vi "JoystickToPoint.vi"(8 "Yw":dbl, 9 "Xw":dbl, 11 "JoystickIn":i32[](array[numeric])) -> (2 "y":dbl, 3 "x":dbl)   [LabVIEW 2013, in "ProcessorHelperFunctions.lvlib"]
uses:
  ProcessorHelperFunctions.lvlib
  <vilib>/Analysis/coordinate.llb/Angle Range (Degree).ctl
  <vilib>/Analysis/coordinate.llb/Angle Rotation (scalar).vi
  <vilib>/Analysis/coordinate.llb/Wrap Angle (scalar).vi
  <vilib>/Analysis/NI_AAL_Angle.lvlib
panel:
  in  "Mag Scaler":dbl=1.5
  # "Xw is x distance between the\nwheels on the robot"
  # "Yw is y distance between the\nwheels on the robot"
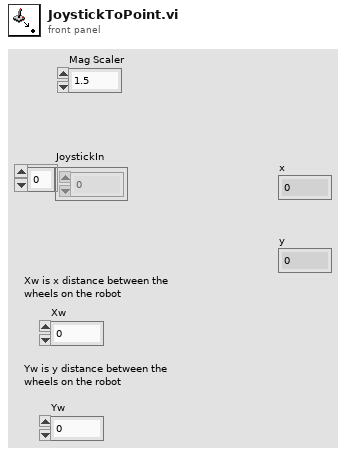
[diagram p1: front panel]
types:
  T1 = typedef "NI_AAL_Angle.lvlib/Angle Range (Degree).ctl" = u16
  T2 = cluster{"JoystickIn[0]":i32, "JoystickIn[1]":i32, "JoystickIn[2]":i32, "JoystickIn[3]":i32, "JoystickIn[4]":i32, "JoystickIn[5]":i32, "JoystickIn[6]":i32, "JoystickIn[7]":i32, "JoystickIn[8]":i32, "JoystickIn[9]":i32}
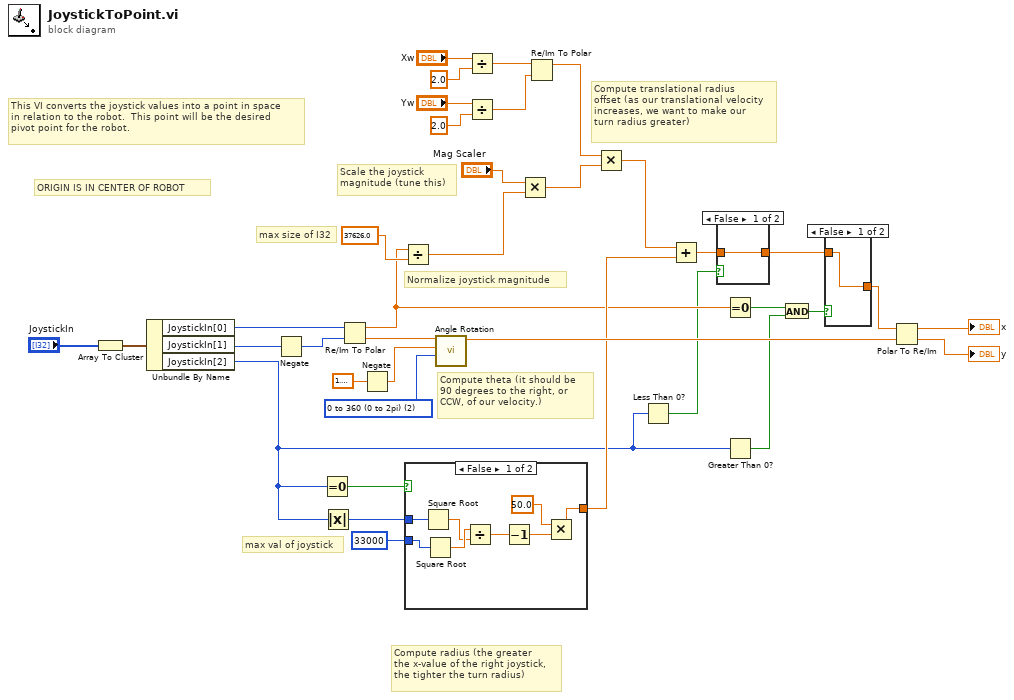
[diagram p0: block diagram]
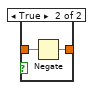
[diagram p2: hidden frame]
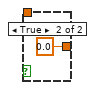
[diagram p3: hidden frame]
diagram:
  w32 = T1 2 items=["none", "-180 to 180 (-pi to pi)", "0 to 360 (0 to 2pi)"] ("rotated angle range")
  # "ORIGIN IS IN CENTER OF ROBOT"
  # "Scale the joystick\nmagnitude (tune this)"
  # "Compute theta (it should be \n90 degrees to the right, or \nCCW, of our velocity.)"
  # "Compute radius (the greater\nthe x-value of the right joystick,\nthe tighter the turn radius)"
  # "Compute translational radius \noffset (as our translational velocity\nincreases, we want to make our\nturn radius greater)"
  # "Normalize joystick magnitude"
  # "max size of I32"
  # "max val of joystick"
  # "This VI converts the joystick values into a point in space\nin relation to the robot.  This point will be the desired\npivot point for the robot."
  n1 = Array To Cluster(array="JoystickIn") -> (cluster=w37:T2)
  n2 = Unbundle By Name(w37) -> ("JoystickIn[0]"=w35:i32, "JoystickIn[1]"=w34:i32, "JoystickIn[2]"=w3:i32)
  n3 = Negate(x=w34) -> (-x=w1:i32)
  n4 = Equal To 0?(x=w3) -> (x = 0?=w30:bool)
  n5 = Absolute Value(x=w3) -> (abs(x)=w6:i32)
  n6 = Re/Im To Polar(2:w1, 3:w35) -> (0:w33:dbl, 1:w9:dbl)
  n7 = Negate(x=1.5707963267948966) -> (-x=w7:dbl)
  n8 = Divide(x=w9, y=37626.0) -> (x/y=w25:dbl)
  n9 = case shown="False" w30 {
    tunnel: 33000 -> [w44 w46]
    tunnel: w6 -> [w45 _]
    tunnel: [w40 w46] -> w21
    frame False {
      n10 = Square Root(x=w45) -> (sqrt(x)=w42:dbl)
      n11 = Square Root(x=w44) -> (sqrt(x)=w43:dbl)
      n12 = Divide(x=w43, y=w42) -> (x/y=w39:dbl)
      n13 = Decrement(x=w39) -> (x-1=w38:dbl)
      n14 = Multiply(x=50.0, y=w38) -> (x*y=w40:dbl)
    }
    frame True {
    }
  }
  n15 = call-poly <vilib>:"Angle Rotation.vi"("rotated angle range"=w32, "counterclockwise rotation"=w7, "angle"=w33) -> ("rotated angle"=w28:dbl)  [unwired: 7 in, 1 out]
  n16 = Divide(x="Xw", y=2.0) -> (x/y=w16:dbl)
  n17 = Divide(x="Yw", y=2.0) -> (x/y=w15:dbl)
  n18 = Multiply(x="Mag Scaler", y=w25) -> (x*y=w24:dbl)
  n19 = Re/Im To Polar(2:w15, 3:w16) -> (1:w23:dbl)  [unwired: 1 out]
  n20 = Multiply(x=w23, y=w24) -> (x*y=w22:dbl)
  n21 = Less Than 0?(x=w3) -> (x < 0?=w2:bool)
  n22 = Add(x=w22, y=w21) -> (x+y=w5:dbl)
  n23 = case shown="False" w2 {
    tunnel: w5 -> [w47 w49]
    tunnel: [w47 w48] -> w4
    frame False {
    }
    frame True {
      n24 = Negate(x=w49) -> (-x=w48:dbl)
    }
  }
  n25 = Equal To 0?(x=w9) -> (x = 0?=w10:bool)
  n26 = Greater Than 0?(x=w3) -> (x > 0?=w11:bool)
  n27 = And(x=w10, y=w11) -> (x .and. y?=w12:bool)
  n28 = case shown="False" w12 {
    tunnel: w4 -> [w50 _]
    tunnel: [w50 0.0] -> w8
    frame False {
    }
    frame True {
    }
  }
  n29 = Polar To Re/Im(2:w28, 3:w8) -> (0:→"y":dbl, 1:→"x":dbl)
